vi "Get_left_right_exp.vi"(8 "error in (no error)":errorcluster, 10 "Data":sgl[][](array[numeric]), 11 "Experiment_merged in":refnum<class "Experiment_merged.lvclass">) -> (0 "error out":errorcluster, 1 "right":sgl[][](array[numeric]), 2 "left":sgl[][](array[numeric]), 3 "Experiment_merged out":refnum<class "Experiment_merged.lvclass">)   [LabVIEW 2018, in "Experiment_merged.lvclass"]
uses:
  Experiment_merged.lvclass
  C:/Users/Sergey Denisov/Documents/REPS/TRANCON/Classes/Experiments/Experiment.lvclass
  Experiment.lvclass
panel:
  in  "Temp":bool=TRUE
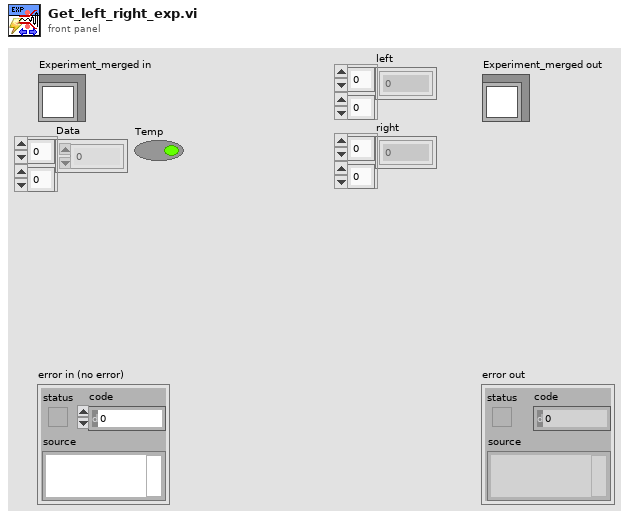
[diagram p1: front panel]
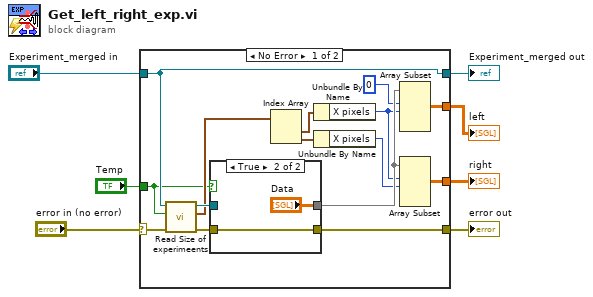
[diagram p0: block diagram]
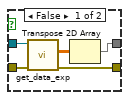
[diagram p2: hidden frame]
diagram:
  n1 = case shown="No Error" "error in (no error)" {
    selector: "error in (no error)" -> [w19 w31]
    tunnel: [w18 w31] -> w6
    tunnel: [w22 w30] -> w4
    tunnel: "Experiment_merged in" -> [w22 w30]
    tunnel: "Temp" -> [w8 _]
    tunnel: [w16 _] -> w2
    tunnel: [w15 _] -> w1
    frame No Error {
      n2 = call-dynamic "Read Size of experimeents.vi"("error in (no error)"=w19, "Temp"=w8, "Experiment_merged in"=w22) -> ("error out"=w20:errorcluster, "Size of experimeents"=w14:cluster{"X pixels":i32, "Y pixels":i32}[], "Experiment_merged out"=w21:refnum<class "Experiment_merged.lvclass">)  [unwired: 6 in]
      n3 = case shown="True" w8 {
        tunnel: w21 -> [w27 _]
        tunnel: w20 -> [w26 w29]
        tunnel: [w25 w29] -> w18
        tunnel: [w23 "Data"] -> w17
        frame False {
          n4 = call "get_data_exp.vi"("error in (no error)"=w26, "Experiment.lvclass in"=w27) -> ("error out"=w25:errorcluster, "Data"=w24:sgl[][])  [unwired: 7 in, 1 out]
          n5 = Transpose 2D Array(2D array=w24) -> (transposed array=w23:sgl[][])
        }
        frame True {
        }
      }
      n6 = Index Array(array=w14) -> (element #1=w13:cluster{"X pixels":i32, "Y pixels":i32}, element #2=w12:cluster{"X pixels":i32, "Y pixels":i32})  [unwired: 2 in]
      n7 = Unbundle By Name(w13) -> ("X pixels"=w10:i32)
      n8 = Unbundle By Name(w12) -> ("X pixels"=w9:i32)
      n9 = Array Subset(array=w17, index (row)=0 ("index"), length (row)=w10) -> (w16:sgl[][])  [unwired: 2 in]
      n10 = Array Subset(array=w17, index (row)=w10, length (row)=w9) -> (w15:sgl[][])  [unwired: 2 in]
    }
    frame Error {
    }
  }
  "error out" <- w6
  "Experiment_merged out" <- w4
  "left" <- w2
  "right" <- w1
